vi "Globa manula or auto mode.vi"() -> ()   [LabVIEW 2019]
panel:
  out "MANULA OR AUTO MODE":bool
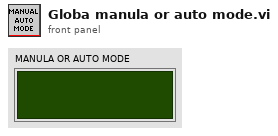
[diagram p1: front panel]
diagram:
